vi "User Dynamic (multiple).vi"(7 "User.lvclass":refnum<class "User.lvclass">, 8 "error in (no error)":errorcluster, 11 "XY-data":cluster{"X-array":dbl[], "Y-array":dbl[]}[](array[cluster]) {"Y-array" format="%.2p"; "X-array" format="%.2p"}) -> (0 "error out":errorcluster, 3 "XY-data out":cluster{"X-array":dbl[], "Y-array":dbl[]}[](array[cluster]) {"Y-array" format="%.2p"; "X-array" format="%.2p"})   [LabVIEW 2019, in "User.lvclass"]
uses:
  User.lvclass
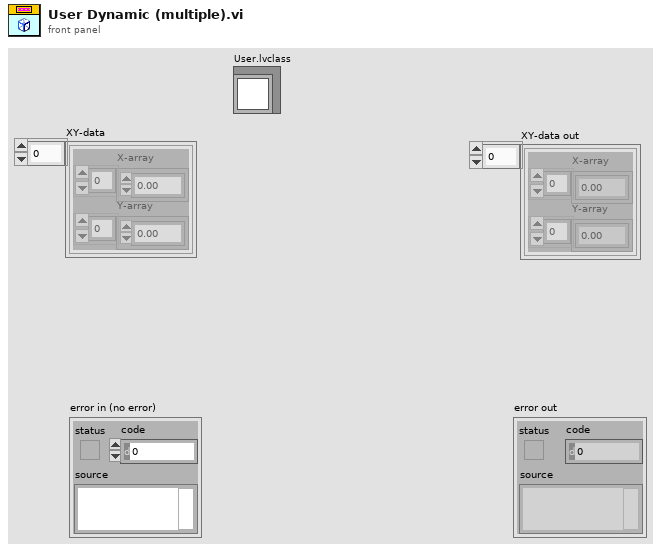
[diagram p1: front panel]
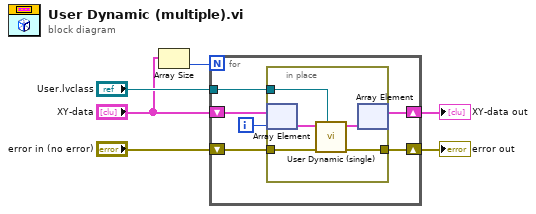
[diagram p0: block diagram]
diagram:
  n1 = Array Size(array="XY-data") -> (size(s)=w3:i32)
  n2 = for {
    N: w3 -> [_]
    tunnel: "User.lvclass" -> [w12]
    shift-right: [w11] -> w1
    shift-left: "XY-data" -> [w7]
    shift-right: [w8] -> w5
    shift-left: "error in (no error)" -> [w9]
    i -> [w10]
    n3 = in-place {
      in-place-border: w12 -> [w13]
      in-place-border: w9 -> [w15]
      in-place-border: [w14] -> w8
      n4 = in-place-array #1(w7, w10) -> (w17:cluster{"X-array":dbl[], "Y-array":dbl[]})
      n5 = call-dynamic "User Dynamic (single).vi"("User.lvclass"=w13, "error in (no error)"=w15, "XY-data"=w17) -> ("error out"=w14:errorcluster, "XY-data out"=w16:cluster{"X-array":dbl[], "Y-array":dbl[]})  [unwired: 7 in]
      n6 = in-place-array #1(w16) -> (w11:cluster{"X-array":dbl[], "Y-array":dbl[]}[])  [unwired: 1 out]
    }
  }
  "error out" <- w5
  "XY-data out" <- w1
